vi "Multi Serial Number Dialog.vi"() -> (3 "Serial Numbers":string[](array[string]))   [LabVIEW 2013]
uses:
  <instrlib>/Driver Simulation/Fixture.lvlib
panel:
  out "error out":errorcluster
  in  "Serial Numbers to Test":string[](array[combo]) caption="Select Serial Numbers to test"
  in  "OK":bool
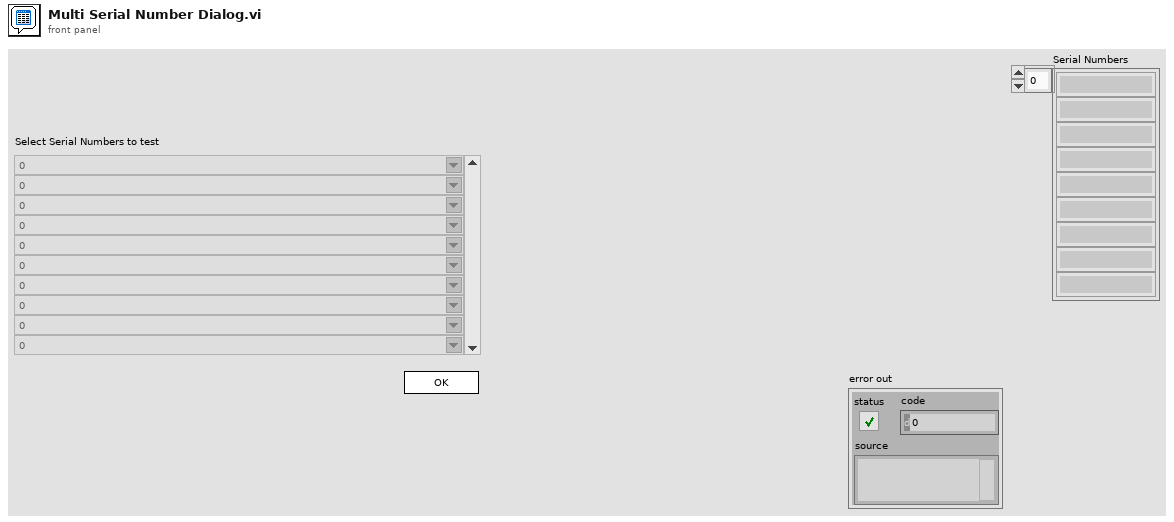
[diagram p1: front panel]
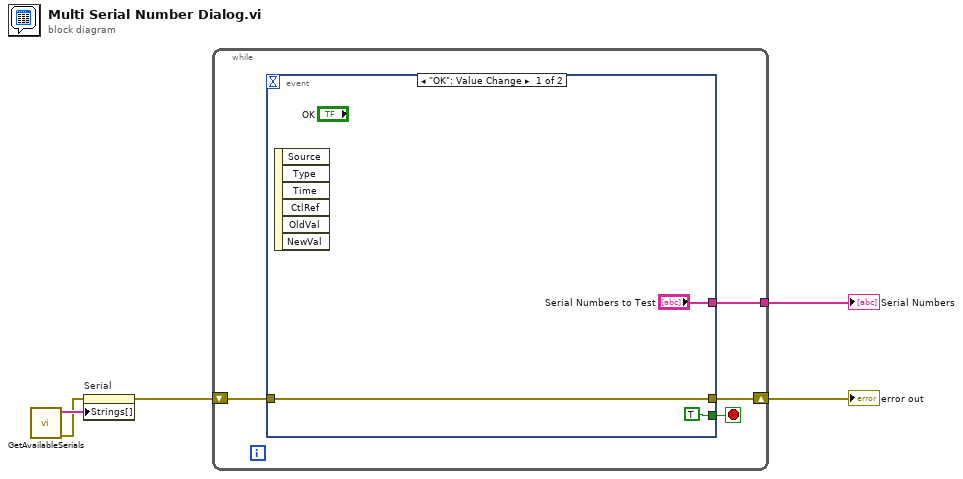
[diagram p0: block diagram]
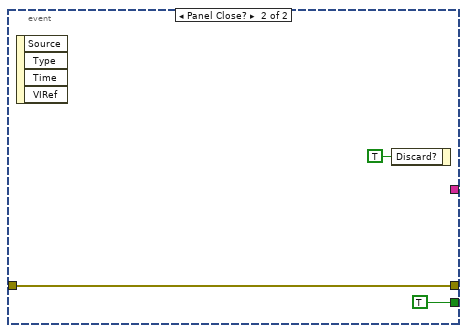
[diagram p2: hidden frame]
diagram:
  n1 = call <instrlib>:"GetAvailableSerials.vi"() -> ("error out"=w3:errorcluster, "serialNumbers"=w4:string[])  [unwired: 10 in]
  n2 = property on="Serial" class="CmbBox"(error in=w3, "Strings[]"=w4) -> (error out=w2:errorcluster)  [unwired: 1 in, 1 out]
  n3 = while {
    tunnel: [w8] -> w5
    shift-right: [w7] -> w1
    shift-left: w2 -> [w6]
    stop <- w9 stop-if-true
    n4 = event shown="[0] \"OK\": Value Change" {
      selector: _ -> [_ _]
      dyn-events: _ -> [_ _]
      timeout: _ -> [_ _]
      tunnel: [TRUE ("OK") TRUE ("OK")] -> w9
      tunnel: ["Serial Numbers to Test" _] -> w8
      tunnel: [w10 w13] -> w7
      tunnel: w6 -> [w10 w13]
      event "OK": Value Change {
        n5 = event-data() -> ()  [unwired: 1 in, 6 out]
      }
      event Panel Close? {
        n6 = event-data() -> ()  [unwired: 1 in, 4 out]
        n7 = event-data("Discard?"=TRUE) -> ()  [unwired: 1 in, 1 out]
      }
    }
  }
  "Serial Numbers" <- w5
  "error out" <- w1
